vi "ReadExpFile.vi"(2 "ExpFilePath":path=path "C:/Data/Matias/NewSoft_test/201707071638.h5") -> (0 "Exp_params":T3 {"File Ref list" format="%.0x"}, 1 "WorkFilePath":path)   [LabVIEW 2013]
uses:
  <vilib>/addons/h5labview2/file/H5Fmode.ctl
  <vilib>/addons/h5labview2/base/hid_t.ctl
  <vilib>/addons/h5labview2/attrib/H5Aread.llb/H5Aread.xnode
  <vilib>/addons/h5labview2/base/H5Equery.vi
  <vilib>/addons/h5labview2/base/lib_path.vi
  fpga-bitfile-ref.ctl
  <vilib>/addons/h5labview2/dataset/H5Dread.llb/H5Dread.xnode
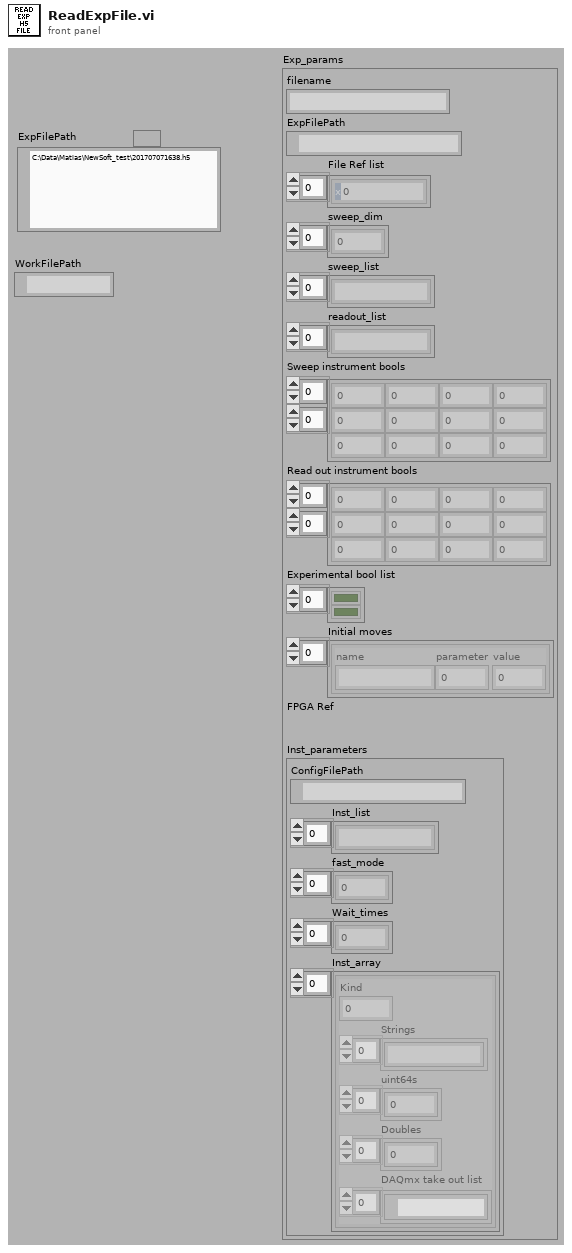
[diagram p1: front panel]
types:
  T1 = typedef "hid_t.ctl" = i32
  T2 = typedef "fpga-bitfile-ref.ctl" = refnum<k20>
  T3 = cluster{"filename":string, "ExpFilePath":path, "File Ref list":T1[], "sweep_dim":u64[], "sweep_list":string[], "readout_list":string[], "Sweep instrument bools":u64[][], "Read out instrument bools":u64[][], "Experimental bool list":bool[], "Initial moves":cluster{"name":string, "parameter":u64, "value":dbl}[], "FPGA Ref":T2, "Inst_parameters":cluster{"ConfigFilePath":path, "Inst_list":string[], "fast_mode":u8[], "Wait_times":u64[], "Inst_array":cluster{"Kind":u16, "Strings":string[], "uint64s":u64[], "Doubles":dbl[], "DAQmx take out list":refnum<k21>[]}[]}}
  T4 = cluster{"name":string, "parameter":u64, "value":dbl}[]
  T5 = cluster{"filename":string, "ExpFilePath":path, "File Ref list":T1[], "sweep_dim":u64[], "sweep_list":string[], "readout_list":string[], "Sweep instrument bools":u64[][], "Read out instrument bools":u64[][], "Experimental bool list":bool[], "Initial move":cluster{"Name":string, "kind":u64, "Value":dbl}[], "FPGA Ref":T2, "Inst_parameters":cluster{"ConfigFilePath":path, "Inst_list":string[], "fast_mode":u8[], "Wait_times":u64[], "Inst_array":cluster{"Kind":u16, "Strings":string[], "uint64s":u64[], "Doubles":dbl[], "DAQmx take out list":refnum<k21>[]}[]}}
  T6 = typedef "H5F.lvlib/H5Fmode.ctl" = enum16{"read-only", "read-write", "overwrite", "create new", "open or create"}
  T7 = cluster{"ConfigFilePath":path, "Inst_list":string[], "fast_mode":u64[], "Wait_times":u64[], "Inst_array":cluster{"Kind":u16, "Strings":string[], "uint64s":u64[], "Doubles":dbl[], "DAQmx take out list":refnum<k21>[]}[]}
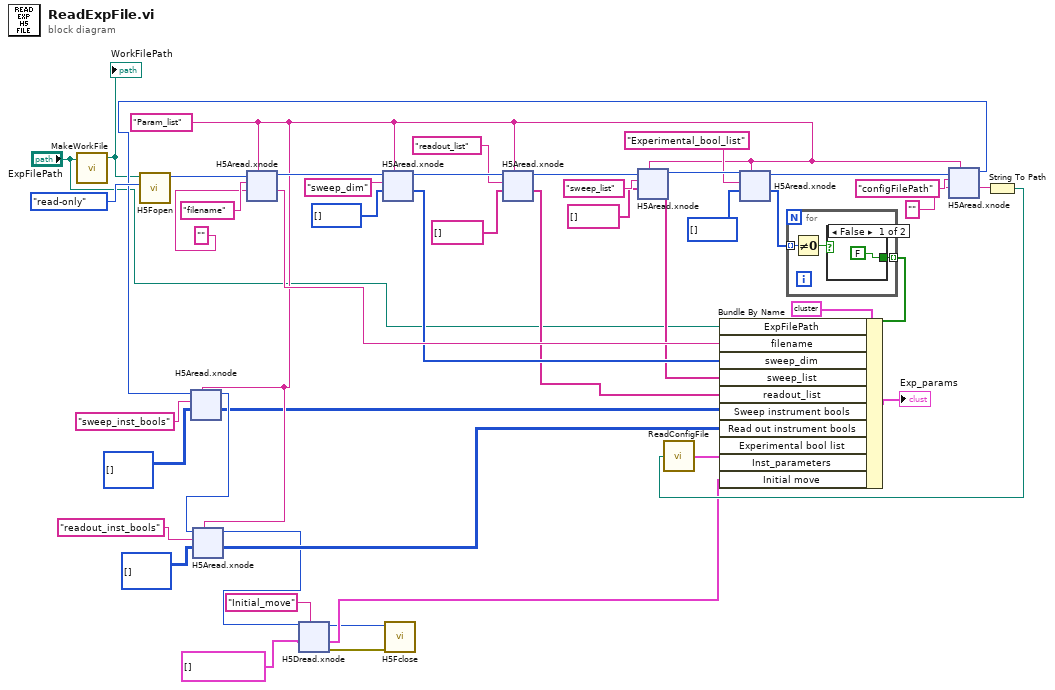
[diagram p0: block diagram]
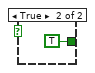
[diagram p2: hidden frame]
diagram:
  w17 = "Param_list"
  n1 = call "MakeWorkFile.vi"("ExpFilePath"="ExpFilePath") -> ("WorkFilePath"=w4:path)  [unwired: 4 in]
  "WorkFilePath" <- w4
  n2 = call <vilib>:"H5Fopen.vi"("mode (read-only)"=H5Fmode."read-only" ("mode"), "path"=w4) -> ("ref out"=w46:T1)  [unwired: 8 in, 1 out]
  n3 = xnode "H5Aread.xnode"("object name"=w17, "default"="", "attrib name"="filename", "ref in"=w46) -> ("data"=w35:string, "ref out"=w43:T1)  [unwired: 2 in, 2 out]
  n4 = xnode "H5Aread.xnode"("object name"=w17, "default"=u64[] [], "attrib name"="sweep_dim", "ref in"=w43) -> ("data"=w34:u64[], "ref out"=w32:T1)  [unwired: 2 in, 2 out]
  n5 = xnode "H5Aread.xnode"("object name"=w17, "default"=string[] [] ("readout_list"), "attrib name"="readout_list", "ref in"=w32) -> ("data"=w28:string[], "ref out"=w31:T1)  [unwired: 2 in, 2 out]
  n6 = xnode "H5Aread.xnode"("object name"=w17, "default"=string[] [], "attrib name"="sweep_list", "ref in"=w31) -> ("data"=w33:string[], "ref out"=w27:T1)  [unwired: 2 in, 2 out]
  n7 = xnode "H5Aread.xnode"("object name"=w17, "default"=u8[] [], "attrib name"="Experimental_bool_list", "ref in"=w27) -> ("data"=w20:u8[], "ref out"=w26:T1)  [unwired: 2 in, 2 out]
  n8 = for {
    tunnel: w20 -> [w49] mode=indexing
    tunnel: [w48] -> w19 mode=indexing
    n9 = Not Equal To 0?(x=w49) -> (x != 0?=w50:bool)
    n10 = case shown="False" w50 {
      tunnel: [FALSE TRUE] -> w48
      frame False {
      }
      frame True {
      }
    }
  }
  n11 = xnode "H5Aread.xnode"("object name"=w17, "default"="", "attrib name"="configFilePath", "ref in"=w26) -> ("data"=w36:string, "ref out"=w22:T1)  [unwired: 2 in, 2 out]
  n12 = xnode "H5Aread.xnode"("object name"=w17, "default"=u64[][] [], "attrib name"="sweep_inst_bools", "ref in"=w22) -> ("data"=w12:u64[][], "ref out"=w16:T1)  [unwired: 2 in, 2 out]
  n13 = xnode "H5Aread.xnode"("object name"=w17, "default"=u64[][] [], "attrib name"="readout_inst_bools", "ref in"=w16) -> ("data"=w11:u64[][], "ref out"=w8:T1)  [unwired: 2 in, 2 out]
  n14 = xnode "H5Dread.xnode"("dataset name (this)"="Initial_move", "default"=T4 [] ("Initial move"), "ref in"=w8) -> ("error out"=w1:errorcluster, "data"=w7:T4, "ref out"=w2:T1)  [unwired: 3 in, 1 out]
  n15 = call <vilib>:"H5Fclose.vi"("error in (no error)"=w1, "ref"=w2) -> ()  [unwired: 9 in, 1 out]
  n16 = String To Path(string=w36) -> (path=w23:path)
  n17 = call "ReadConfigFile.vi"("ConfigFilePath"=w23) -> ("Inst_parameters"=w24:T7)
  n18 = Bundle By Name(cluster=T5 {"filename"="", "ExpFilePath"=path "", "File Ref list"=[], "sweep_dim"=[5], "sweep_list"=["0:1"], "readout_list"=["ADC0", "ADC1"], "Sweep instrument bools"=[], "Read out instrument bools"=[], "Experimental bool list"=[TRUE, TRUE], "Initial move"=[], "FPGA Ref"=refnum, "Inst_parameters"={"ConfigFilePath"=path "", "Inst_list"=["ADC", "0:0", "0:1", "0:2", "0:3", "0:4", "0:5", "0:6", "0:7", "2:0", "2:1", "2:2", "2:3", "2:4", "2:5", "2:6", "2:7", "fast_sequence"], "fast_mode"=[1, 0], "Wait_times"=[10, 10, 10, 10], "Inst_array"=[{"Kind"=0, "Strings"=["ADC", "", "V", "ADC0;ADC1", "V;V"], "uint64s"=[10, 2, 250000, 1, 100, 10106, 1000000], "Doubles"=[1.0], "DAQmx take out list"=[]}, {"Kind"=4, "Strings"=["0:0", "10.0.0.2", "V"], "uint64s"=[0, 0], "Doubles"=[0.30000001192092896, -2.0, 2.0, -1.0], "DAQmx take out list"=[]}, {"Kind"=4, "Strings"=["0:1", "10.0.0.2", "V"], "uint64s"=[0, 1], "Doubles"=[0.30000001192092896, -2.0, 2.0, -1.0], "DAQmx take out list"=[]}, {"Kind"=4, "Strings"=["0:2", "10.0.0.2", "V"], "uint64s"=[0, 2], "Doubles"=[0.30000001192092896, -2.0, 2.0, -1.0], "DAQmx take out list"=[]}, {"Kind"=4, "Strings"=["0:3", "10.0.0.2", "V"], "uint64s"=[0, 3], "Doubles"=[0.30000001192092896, -2.0, 2.0, -1.0], "DAQmx take out list"=[]}, {"Kind"=4, "Strings"=["0:4", "10.0.0.2", "V"], "uint64s"=[0, 4], "Doubles"=[0.30000001192092896, -2.0, 2.0, -1.0], "DAQmx take out list"=[]}, {"Kind"=4, "Strings"=["0:5", "10.0.0.2", "V"], "uint64s"=[0, 5], "Doubles"=[0.30000001192092896, -2.0, 2.0, -1.0], "DAQmx take out list"=[]}, {"Kind"=4, "Strings"=["0:6", "10.0.0.2", "V"], "uint64s"=[0, 6], "Doubles"=[0.30000001192092896, -2.0, 2.0, -1.0], "DAQmx take out list"=[]}, {"Kind"=4, "Strings"=["0:7", "10.0.0.2", "V"], "uint64s"=[0, 7], "Doubles"=[0.30000001192092896, -2.0, 2.0, -1.0], "DAQmx take out list"=[]}, {"Kind"=4, "Strings"=["2:0", "10.0.0.2", "V"], "uint64s"=[2, 0], "Doubles"=[0.30000001192092896, -2.0, 2.0, -1.0], "DAQmx take out list"=[]}, {"Kind"=4, "Strings"=["2:1", "10.0.0.2", "V"], "uint64s"=[2, 1], "Doubles"=[0.30000001192092896, -2.0, 2.0, -1.0], "DAQmx take out list"=[]}, {"Kind"=4, "Strings"=["2:2", "10.0.0.2", "V"], "uint64s"=[2, 2], "Doubles"=[0.30000001192092896, -2.0, 2.0, -1.0], "DAQmx take out list"=[]}, {"Kind"=4, "Strings"=["2:3", "10.0.0.2", "V"], "uint64s"=[2, 3], "Doubles"=[0.30000001192092896, -2.0, 2.0, -1.0], "DAQmx take out list"=[]}, {"Kind"=4, "Strings"=["2:4", "10.0.0.2", "V"], "uint64s"=[2, 4], "Doubles"=[0.30000001192092896, -2.0, 2.0, -1.0], "DAQmx take out list"=[]}, {"Kind"=4, "Strings"=["2:5", "10.0.0.2", "V"], "uint64s"=[2, 5], "Doubles"=[0.30000001192092896, -2.0, 2.0, -1.0], "DAQmx take out list"=[]}, {"Kind"=4, "Strings"=["2:6", "10.0.0.2", "V"], "uint64s"=[2, 6], "Doubles"=[0.30000001192092896, -2.0, 2.0, -1.0], "DAQmx take out list"=[]}, {"Kind"=4, "Strings"=["2:7", "10.0.0.2", "V"], "uint64s"=[2, 7], "Doubles"=[0.30000001192092896, -2.0, 2.0, -1.0], "DAQmx take out list"=[]}, {"Kind"=9, "Strings"=["fast_sequence", "10.0.0.2", "V"], "uint64s"=[44439, 300, 200, 0, 0, 1, 2, 3, 4, 5, 6, 7, 16, 17, 18, 19, 20, 21, 22, 23], "Doubles"=[0.5, -0.5, -1.0, -1.0], "DAQmx take out list"=[]}]}} ("Exp_params 2"), "ExpFilePath"="ExpFilePath", "filename"=w35, "sweep_dim"=w34, "sweep_list"=w33, "readout_list"=w28, "Sweep instrument bools"=w12, "Read out instrument bools"=w11, "Experimental bool list"=w19, "Inst_parameters"=w24, "Initial move"=w7) -> (→"Exp_params":T5)
